vi "main-20220126.vi"   [LabVIEW 2019]
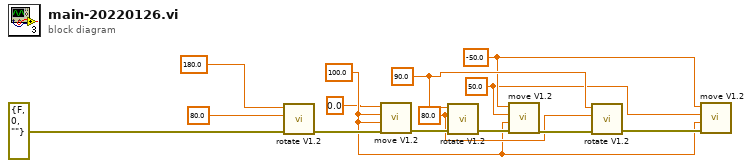
[diagram p0: block diagram]
diagram:
  w2 = 50.0 ("Y")
  w3 = -50.0 ("X")
  w7 = 80.0 ("speed")
  w6 = 90.0 ("degree")
  w4 = 100.0 ("X")
  n1 = call "rotate V1.2.vi"("error in (no error)"=errorcluster {"status"=FALSE, "code"=0, "source"=""}, "speed"=80.0, "degree"=180.0) -> ("error out"=w13:errorcluster)  [unwired: 8 in]
  n2 = call "move V1.2.vi"("error in (no error)"=w13, "RPM"=w4, "Y"=w4, "X"=0.0) -> ("error out"=w14:errorcluster)  [unwired: 7 in]
  n3 = call "rotate V1.2.vi"("error in (no error)"=w14, "speed"=w7, "degree"=w6) -> ("error out"=w9:errorcluster)  [unwired: 8 in]
  n4 = call "move V1.2.vi"("error in (no error)"=w9, "RPM"=w4, "Y"=w2, "X"=w3) -> ("error out"=w8:errorcluster)  [unwired: 7 in]
  n5 = call "rotate V1.2.vi"("error in (no error)"=w8, "speed"=w7, "degree"=w6) -> ("error out"=w5:errorcluster)  [unwired: 8 in]
  n6 = call "move V1.2.vi"("error in (no error)"=w5, "RPM"=w4, "Y"=w2, "X"=w3) -> ()  [unwired: 7 in, 1 out]
